vi "version_to_string.vi"(8 "error in (no error)":errorcluster, 11 "version":T1) -> (0 "error out":errorcluster, 3 "version":string)   [LabVIEW 2015, in "lv-builder-default.lvlib"]
uses:
  lv-builder-default.lvlib
  public/_controls/version.ctl
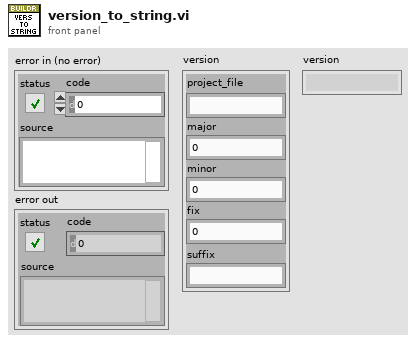
[diagram p1: front panel]
types:
  T1 = typedef "lv-builder-default.lvlib/version.ctl" = cluster{"project_file":string, "major":u32, "minor":u32, "fix":u32, "suffix":string}
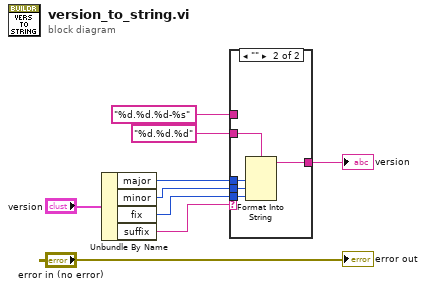
[diagram p0: block diagram]
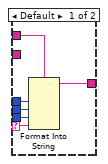
[diagram p2: hidden frame]
diagram:
  n1 = Unbundle By Name("version") -> ("major"=w7:u32, "minor"=w5:u32, "fix"=w4:u32, "suffix"=w2:string)
  n2 = case shown="\"\"" w2 {
    selector: w2 -> [w10 _]
    tunnel: w7 -> [w15 w20]
    tunnel: [w14 w19] -> w6
    tunnel: w5 -> [w13 w18]
    tunnel: w4 -> [w12 w17]
    tunnel: "%d.%d.%d-%s" ("format string") -> [w11 _]
    tunnel: "%d.%d.%d" ("format string") -> [_ w16]
    frame Default {
      n3 = Format Into String(format string=w11, w15, w13, w12, w10) -> (resulting string=w14:string)  [unwired: 2 in, 1 out]
    }
    frame "" {
      n4 = Format Into String(format string=w16, w20, w18, w17) -> (resulting string=w19:string)  [unwired: 2 in, 1 out]
    }
  }
  "version" <- w6
  "error out" <- "error in (no error)"
